vi "NIMS_DF_fir_minphase.vi"(11 "b1":dbl[](array[numeric])) -> (0 "error":i32, 3 "b2":dbl[](array[numeric]))   [LabVIEW 2017, in "NI_DigFilter_MathScript.lvlib"]
uses:
  <vilib>/addons/Digital Filter Design/NI_DigFilter_MathScript.lvlib
  <vilib>/addons/Digital Filter Design/NI_DigFilterLicensed.lvlib
panel:
  in  "reserved":i32=-1
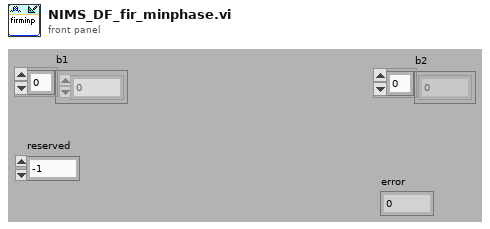
[diagram p1: front panel]
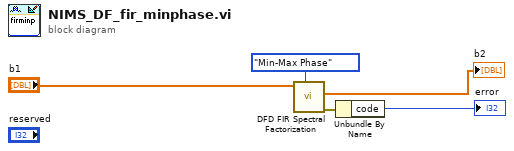
[diagram p0: block diagram]
diagram:
  n1 = call <vilib>:"DFD FIR Spectral Factorization.vi"("method (Min-Max Phase)"=enum16{"Min-Max Phase", "Linear Phase"}."Min-Max Phase", "H(n)"="b1") -> ("error out"=w4:errorcluster, "H(n) 1"=→"b2":dbl[])  [unwired: 1 in, 7 out]
  n2 = Unbundle By Name(w4) -> ("code"=→"error":i32)
